vi "find peak action stack.vi"(7 "stack action":T2, 8 "find peak action list":T1[](array[typedef]), 9 "find fit action":T1=enum."bbb", 11 "command stack":T1[](array[typedef])) -> (1 "find fit action out":T1=enum."bbb", 2 "stack is empty ?":bool, 3 "command stack out":T1[](array[typedef]))   [LabVIEW 2015]
uses:
  stack action -- control.ctl
  find peak action.ctl
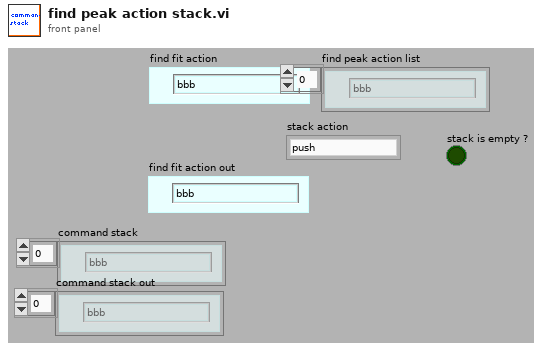
[diagram p1: front panel]
types:
  T1 = typedef "find peak action.ctl" = enum16{"empty", "-find center", "-mapping", "fit", "-shake it one", "bbb", "-update pond", "move z(center)", "move z(inf)", "update pond", "fancy fit one", "fragment window moves", "-shake it two", "fancy fit two", "pm fit"}
  T2 = typedef "stack action -- control.ctl" = enum16{"push", "pop", "check", "init"}
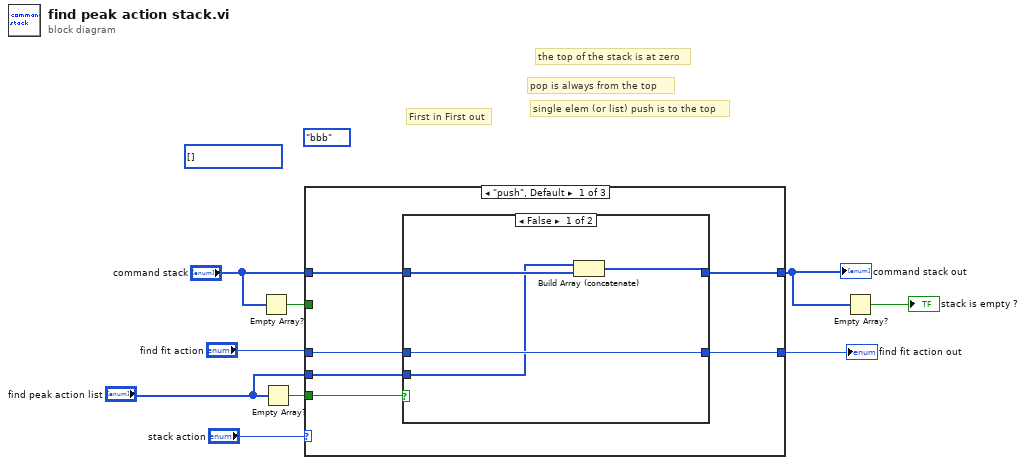
[diagram p0: block diagram]
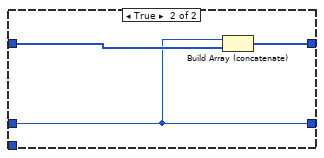
[diagram p2: hidden frame]
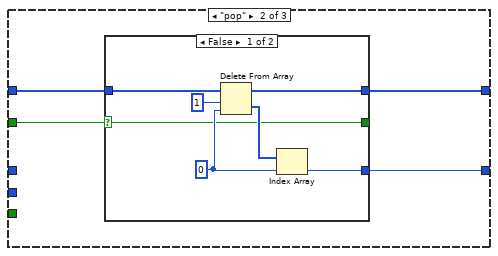
[diagram p3: hidden frame]
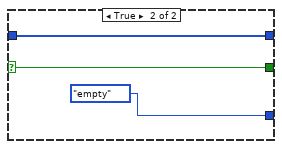
[diagram p4: hidden frame]
diagram:
  (unwired) find_peak_action."bbb" ("cursor window action")
  (unwired) T1[] [] items=["empty", "-find center", "-mapping", "fit", "-shake it one", "bbb", "-update pond", "move z(center)", "move z(inf)", "update pond", "fancy fit one", "fragment window moves", "-shake it two", "fancy fit two", "pm fit"] ("command stack")
  # "single elem (or list) push is to the top"
  # "pop is always from the top"
  # "First in First out"
  # "the top of the stack is at zero"
  n1 = Empty Array?(array="command stack") -> (empty?=w8:bool)
  n2 = Empty Array?(array="find peak action list") -> (empty?=w7:bool)
  n3 = case shown="\"push\", Default" "stack action" {
    tunnel: [w15 w26 w37] -> w2
    tunnel: "command stack" -> [w14 w25 w37]
    tunnel: w8 -> [_ w24 _]
    tunnel: [w10 w23 w38] -> w4
    tunnel: "find fit action" -> [w13 _ w38]
    tunnel: w7 -> [w12 _ _]
    tunnel: "find peak action list" -> [w11 _ _]
    frame "push", Default {
      n4 = case shown="False" w12 {
        tunnel: [w16 w22] -> w15
        tunnel: w14 -> [w18 w21]
        tunnel: w13 -> [w19 w20]
        tunnel: w11 -> [w17 _]
        tunnel: [w19 w20] -> w10
        frame False {
          n5 = Build Array (concatenate)(w17, w18) -> (w16:T1[])
        }
        frame True {
          n6 = Build Array (concatenate)(w20, w21) -> (w22:T1[])
        }
      }
    }
    frame "pop" {
      n7 = case shown="False" w24 {
        selector: w24 -> [w27 w35]
        tunnel: [w33 w36] -> w26
        tunnel: w25 -> [w32 w36]
        tunnel: [w28 find_peak_action."empty" ("cursor window action")] -> w23
        tunnel: [w27 w35] -> _
        frame False {
          w29 = 0
          n8 = Delete From Array(array=w32, length=1, index=w29) -> (deleted portion=w30:T1[], array with subset deleted=w33:T1[])
          n9 = Index Array(array=w30, index=w29) -> (element=w28:T1)
        }
        frame True {
        }
      }
    }
    frame "check" {
    }
  }
  "find fit action out" <- w4
  "command stack out" <- w2
  n10 = Empty Array?(array=w2) -> (empty?=→"stack is empty ?":bool)
